vi "PortInit - 9600.vi"(1 "PortNumber Z":i32=1 caption="PortNumber") -> (0 "Done":bool=TRUE)   [LabVIEW 2015]
panel:
  in  "Baud rate Z":u32=9600
  # "Port Number 0=COM1"
  # "Initialize Serial Port. for Z axis\nDefault setting is 9600/8N1/None."
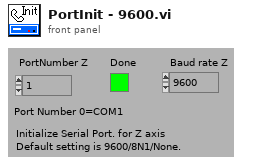
[diagram p1: front panel]
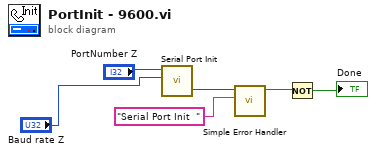
[diagram p0: block diagram]
diagram:
  n1 = call <vilib>:"Serial Port Init.vi"("baud rate"="Baud rate Z", "port number"="PortNumber Z") -> ("error code"=w5:i32)  [unwired: 5 in]
  n2 = call <vilib>:"Simple Error Handler.vi"("error code (no error:0)"=w5, "error source (\" \")"="Serial Port Init  ") -> ("error?"=w4:bool)  [unwired: 2 in, 5 out]
  n3 = Not(x=w4) -> (.not. x?=→"Done":bool)
